vi "Arduino.vi"(0 "Serial Com":refnum<visa-resource-name>, 2 "Function":string(combo), 11 "error in (no error)":errorcluster) -> (4 "Serial Out":refnum<visa-resource-name>, 8 "result":string, 13 "ok?":bool, 15 "error out":errorcluster)   [LabVIEW 2015]
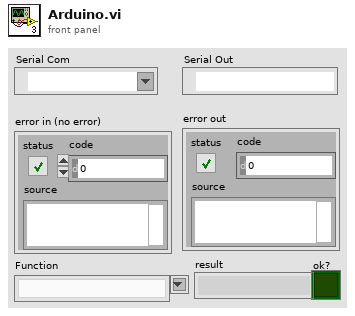
[diagram p1: front panel]
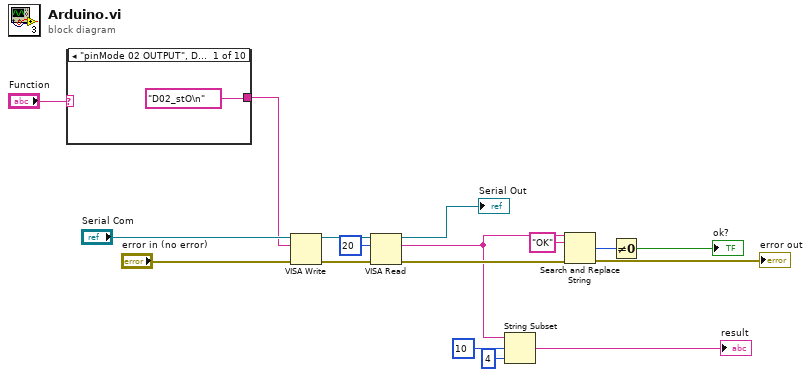
[diagram p0: block diagram]
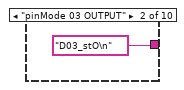
[diagram p2: hidden frame]
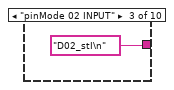
[diagram p3: hidden frame]
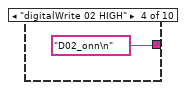
[diagram p4: hidden frame]
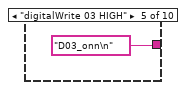
[diagram p5: hidden frame]
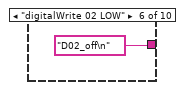
[diagram p6: hidden frame]
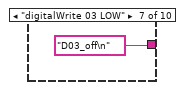
[diagram p7: hidden frame]
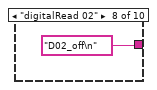
[diagram p8: hidden frame]
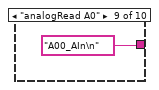
[diagram p9: hidden frame]
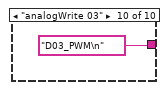
[diagram p10: hidden frame]
diagram:
  n1 = case shown="\"pinMode 02 OUTPUT\", Default" "Function" {
    tunnel: ["D02_stO\n" ("write buffer") "D03_stO\n" ("write buffer") "D02_stI\n" ("write buffer") "D02_onn\n" ("write buffer") "D03_onn\n" ("write buffer") "D02_off\n" ("write buffer") "D03_off\n" ("write buffer") "D02_off\n" ("write buffer") "A00_AIn\n" ("write buffer") "D03_PWM\n" ("write buffer")] -> w3
    frame "pinMode 02 OUTPUT", Default {
    }
    frame "pinMode 03 OUTPUT" {
    }
    frame "pinMode 02 INPUT" {
    }
    frame "digitalWrite 02 HIGH" {
    }
    frame "digitalWrite 03 HIGH" {
    }
    frame "digitalWrite 02 LOW" {
    }
    frame "digitalWrite 03 LOW" {
    }
    frame "digitalRead 02" {
    }
    frame "analogRead A0" {
    }
    frame "analogWrite 03" {
    }
  }
  n2 = VISA Write(VISA resource name="Serial Com", write buffer=w3, error in (no error)="error in (no error)") -> (VISA resource name out=w16:refnum<visa-resource-name>, error out=w17:errorcluster)  [unwired: 1 out]
  n3 = VISA Read(VISA resource name=w16, byte count=u32 20, error in (no error)=w17) -> (VISA resource name out=→"Serial Out":refnum<visa-resource-name>, read buffer=w8:string, error out=w11:errorcluster)  [unwired: 1 out]
  n4 = String Subset(string=w8, offset (0)=10, length (rest)=4 ("length (rest)")) -> (substring=→"result":string)
  n5 = Search and Replace String(input string=w8, search string="OK", error in=w11) -> (number of replacements=w6:i32, error out=→"error out":errorcluster)  [unwired: 5 in, 2 out]
  n6 = Not Equal To 0?(x=w6) -> (x != 0?=→"ok?":bool)
